vi "CompileSubVIs.vi"(8 "error in":errorcluster, 11 "RasPi Compiler in":refnum<class "RasPi Compiler.lvclass">) -> (0 "error out":errorcluster, 3 "RasPi Compiler out":refnum<class "RasPi Compiler.lvclass">)   [LabVIEW 2014, in "Raspberry Pi Compatible Compiler for LabVIEW.lvlib" / "RasPi Compiler.lvclass"]
uses:
  RasPi Compiler.lvclass
  VI Interpreter/Classes/SubVI/SubVI.lvclass
  RasPi Compiler.lvclass/RasPi Compiler.ctl
  VI Interpreter/Classes/VI Interpreter/VI Interpreter.lvclass
  Python/PythonConverter_BD/PyConvBD.lvclass
  RasPi_Services/MessageBox/MessageBox.lvclass
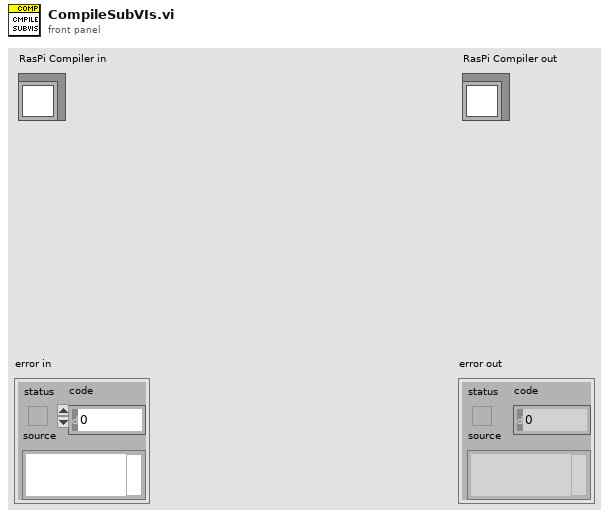
[diagram p1: front panel]
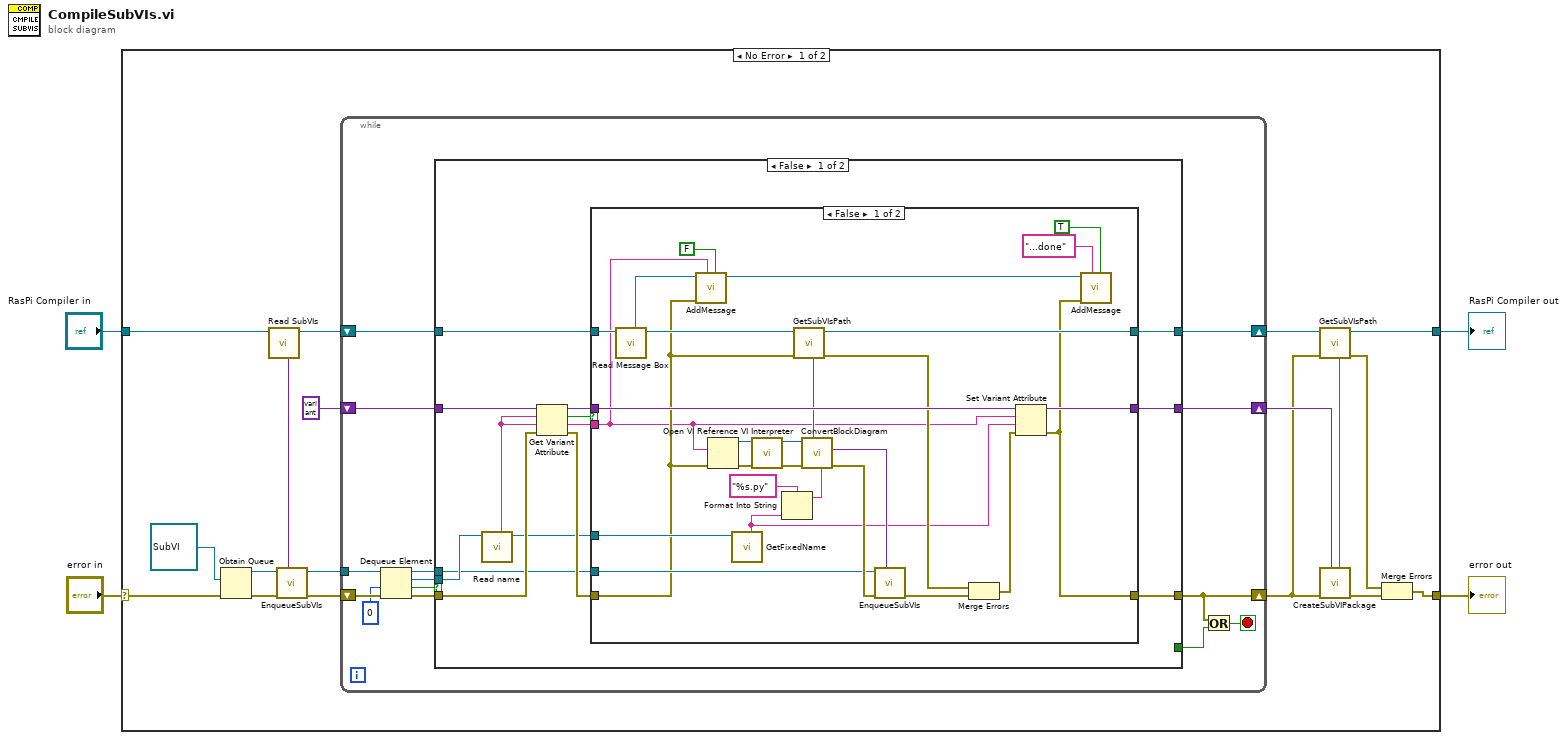
[diagram p0: block diagram]
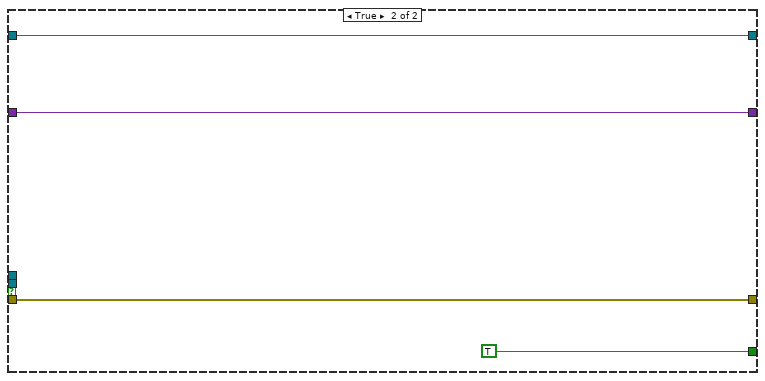
[diagram p3: hidden frame]
diagram:
  n1 = case shown="No Error" "error in" {
    selector: "error in" -> [w19 w87]
    tunnel: [w6 w87] -> w3
    tunnel: [w10 w86] -> w1
    tunnel: "RasPi Compiler in" -> [w21 w86]
    frame No Error {
      n2 = Obtain Queue(element data type=refnum<class "SubVI.lvclass"> refnum ("SubVI.lvclass"), error in (no error)=w19) -> (queue out=w18:refnum<queue>, error out=w17:errorcluster)  [unwired: 3 in, 1 out]
      n3 = call "Read SubVIs.vi"("RasPi Compiler in"=w21) -> ("RasPi Compiler out"=w13:refnum<class "RasPi Compiler.lvclass">, "SubVIs"=w16:variant)  [unwired: 7 in]
      n4 = call "EnqueueSubVIs.vi"("SubVIs"=w16, "error in"=w17, "queue"=w18) -> ("error out"=w14:errorcluster, "queue out"=w15:refnum<queue>)  [unwired: 5 in]
      n5 = while {
        shift-right: [w26] -> w12
        shift-left: variant -> [w29]
        tunnel: w15 -> [w35]
        shift-right: [w27] -> w11
        shift-left: w13 -> [w28]
        shift-right: [w24] -> w8
        shift-left: w14 -> [w36]
        stop <- w23 stop-if-true
        n6 = Dequeue Element(queue=w35, timeout in ms (-1)=0, error in (no error)=w36) -> (queue out=w31:refnum<queue>, element=w30:refnum<class "SubVI.lvclass">, timed out?=w33:bool, error out=w32:errorcluster)
        n7 = case shown="False" w33 {
          tunnel: w32 -> [w50 w82]
          tunnel: w31 -> [w38 _]
          tunnel: w30 -> [w49 _]
          tunnel: w29 -> [w48 w83]
          tunnel: w28 -> [w46 w84]
          tunnel: [_ TRUE] -> w25
          tunnel: [w45 w84] -> w27
          tunnel: [w43 w83] -> w26
          tunnel: [w42 w82] -> w24
          frame False {
            n8 = call-dynamic "Read name.vi"("SubVI in"=w49) -> ("SubVI out"=w37:refnum<class "SubVI.lvclass">, "name"=w40:string)  [unwired: 7 in]
            n9 = Get Variant Attribute(Variant=w48, name=w40, default value (empty Variant)=w40, error in=w50) -> (duplicate Variant=w44:variant, found=w47:bool, value=w39:string, error out=w41:errorcluster)
            n10 = case shown="False" w47 {
              tunnel: w46 -> [w60 w81]
              tunnel: [w66 w81] -> w45
              tunnel: w44 -> [w71 w80]
              tunnel: [w72 w80] -> w43
              tunnel: [w54 w79] -> w42
              tunnel: w41 -> [w57 w79]
              tunnel: w39 -> [w56 _]
              tunnel: w38 -> [w70 _]
              tunnel: w37 -> [w69 _]
              frame False {
                n11 = call "Read Message Box.vi"("RasPi Compiler in"=w60) -> ("RasPi Compiler out"=w59:refnum<class "RasPi Compiler.lvclass">, "Message Box"=w58:refnum<class "MessageBox.lvclass">)  [unwired: 7 in]
                n12 = call "AddMessage.vi"("add newline"=FALSE, "message"=w56, "error in"=w57, "MessageBox in"=w58) -> ("MessageBox out"=w53:refnum<class "MessageBox.lvclass">)  [unwired: 4 in, 1 out]
                n13 = Open VI Reference(vi path=w56, error in (no error)=w57) -> (vi reference=w78:refnum<vi>, error out=w77:errorcluster)  [unwired: 4 in]
                n14 = call-dynamic "GetFixedName.vi"("SubVI in"=w69) -> ("fixed name"=w61:string)  [unwired: 6 in, 2 out]
                n15 = call "VI Interpreter.vi"("error in"=w77, "vi reference"=w78) -> ("error out"=w75:errorcluster, "VI Interpreter out"=w76:refnum<class "VI Interpreter.lvclass">)  [unwired: 8 in]
                n16 = Format Into String(format string="%s.py", w61) -> (resulting string=w68:string)  [unwired: 2 in, 1 out]
                n17 = call "GetSubVIsPath.vi"("error in"=w57, "RasPi Compiler in"=w59) -> ("error out"=w64:errorcluster, "RasPi Compiler out"=w66:refnum<class "RasPi Compiler.lvclass">, "SubVIs path"=w65:path)  [unwired: 5 in]
                n18 = call "ConvertBlockDiagram.vi"("filename"=w68, "Source Directory"=w65, "error in"=w75, "VI Interpreter"=w76) -> ("error out"=w74:errorcluster, "SubVIs"=w73:variant)  [unwired: 3 in, 1 out]
                n19 = call "EnqueueSubVIs.vi"("SubVIs"=w73, "error in"=w74, "queue"=w70) -> ("error out"=w63:errorcluster)  [unwired: 5 in, 1 out]
                n20 = Merge Errors(w64, w63) -> (w62:errorcluster)
                n21 = Set Variant Attribute(Variant=w71, name=w56, value=w61, error in=w62) -> (Variant out=w72:variant, error out=w54:errorcluster)  [unwired: 1 out]
                n22 = call "AddMessage.vi"("add newline"=TRUE, "message"="...done", "error in"=w54, "MessageBox in"=w53) -> ()  [unwired: 4 in, 2 out]
              }
              frame True {
              }
            }
          }
          frame True {
          }
        }
        n23 = Or(x=w24, y=w25) -> (x .or. y?=w23:bool)
      }
      n24 = call "GetSubVIsPath.vi"("error in"=w8, "RasPi Compiler in"=w11) -> ("error out"=w5:errorcluster, "RasPi Compiler out"=w10:refnum<class "RasPi Compiler.lvclass">, "SubVIs path"=w9:path)  [unwired: 5 in]
      n25 = call "CreateSubVIPackage.vi"("SubVIs path"=w9, "SubVIs"=w12, "error in"=w8) -> ("error out"=w7:errorcluster)  [unwired: 6 in]
      n26 = Merge Errors(w5, w7) -> (w6:errorcluster)
    }
    frame Error {
    }
  }
  "error out" <- w3
  "RasPi Compiler out" <- w1
